vi "StepSysIDRealtime.vi"() -> ()   [LabVIEW 2011]
doc: "This VI was generated automatically using the FPGA Wizard. You can modify the VI normally."
uses:
  <vilib>/rvi/interface/nirviMethod/nirviMethod.xnode
  <vilib>/rvi/interface/nirviCloseFPGA/nirviCloseFPGA.xnode
  <vilib>/rvi/interface/nirviOpenFPGA/nirviOpenFPGA.xnode
  SysIDRealtime.lvlib
  <vilib>/rvi/interface/nirviReadWriteControl/nirviReadWriteControl.xnode
  <vilib>/rvi/errors/niLvFpgaAdjustHostInterfaceError.vi
  <vilib>/rvi/interface/Simulation/niFpgaSimulationCallBeginRW.vi
  NiFpgaLv.dll
  <vilib>/Utility/error.llb/Error Cluster From Error Code.vi
  <vilib>/Platform/TimedLoop/XDataNode/XDataNode.xnode
  <vilib>/Platform/TimedLoop/XDataNode/nitl_modes.ctl
  <vilib>/Platform/TimedLoop/XDataNode/XDNodeRunTimeDep.lvlib
  <vilib>/Platform/TimedLoop/XDataNode/wakeup.ctl
  <vilib>/Platform/TimedLoop/XDataNode/timing_clust.ctl
  <vilib>/Analysis/NI_AALBase.lvlib
  <vilib>/FPGAPlugInAG/Dynamic/niLvFpga_Reset_Dynamic.vi
  <vilib>/FPGAPlugInAG/Dynamic/niLvFpga_Run_Dynamic.vi
  <vilib>/FPGAPlugInAG/Dynamic/niLvFpga_Close_Dynamic.vi
  FPGA Bitfiles/PPDControlLab3_FPGATarget_SYSIDFPGA_8751AF80.lvbitx
  SYSID_FPGA.vi
  <vilib>/FPGAPlugInAG/sbRIO-9642/niLvFpga_Open_sbRIO-9642.vi
  <vilib>/rvi/interface/common/dynamic/niFpgaDynamicAddResources.vi
panel:
  out "Amp In":dbl[](graph)
  out "Amp Cpmmand":fxp<+/-,20,5>
  out "Iteration Duration":i64
  out "Position":i32[](graph)
  in  "Control Rate (ticks)":u32=800
  out "error":i32
  out "Waveform Graph":i32[](graph)
  in  "f2":dbl=0.5 format="%0.2f"
  in  "f1":dbl=1.0
  in  "amplitude":dbl=32767.0 format="%0.2f"
  in  "Period (us)":i64=400
  out "Finished Late? [i-1]":bool
  out "quad saved (Port0/DIO0,Port0/DIO1)":cluster{"Position":i32, "Index Count":u16}
  out "quad pos (Port0/DIO0,Port0/DIO1)":i32
  in  "AO (ModB/AO2)":fxp<+/-,20,5>
  in  "AO (ModB/AO1)":fxp<+/-,20,5>
  out "AI (ModA/AI0)":fxp<+/-,26,5> format="%.6g"
  out "Late? Latched":bool
  in  "Local Stop 0":bool
  in  "Start 0":bool
  in  "Loop Rate (Hz)":dbl=70000.0
  out "Calculated Rate (Hz)":dbl
  out "error out":errorcluster
  in  "Global Stop":bool
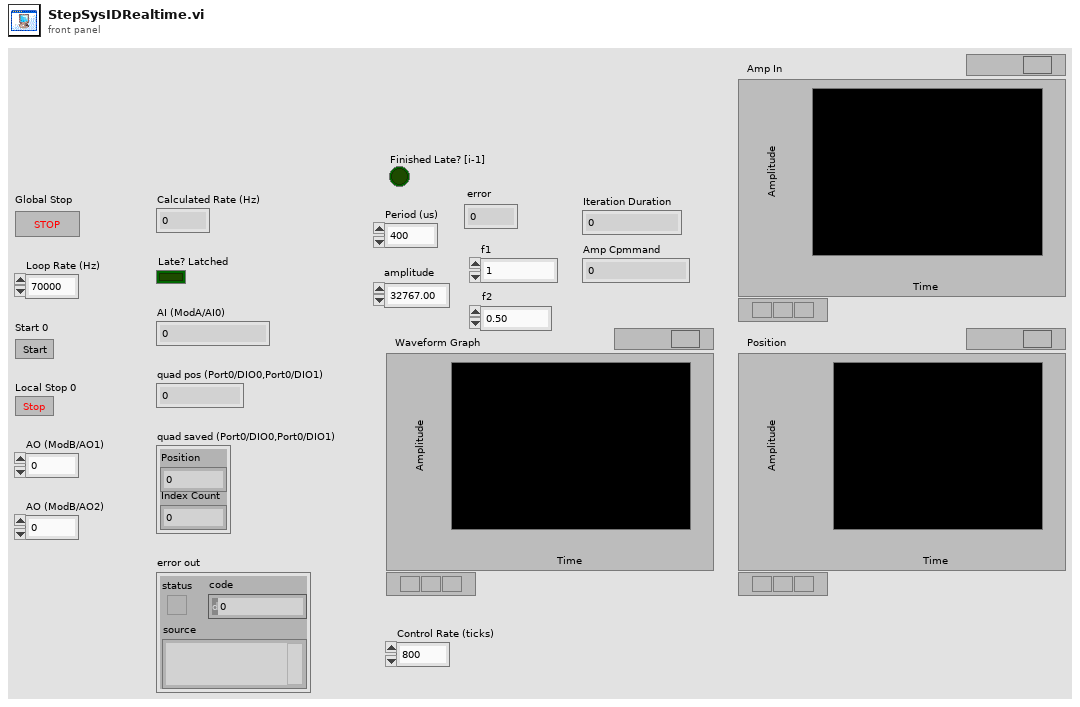
[diagram p1: front panel]
types:
  T1 = typedef "XDNodeRunTimeDep.lvlib/timing_clust.ctl" = cluster{"Expected End [f-1]":u64, "Actual End [f-1]":u64, "Finished Late? [f-1]":bool, "Expected End [i-1]":u64, "Actual End [i-1]":u64, "Finished Late? [i-1]":bool, "Expected Start [i]":u64, "Actual Start [i]":u64, "Expected Start [f]":u64, "Actual Start [f]":u64, "Source Name":string, "Structure Name":string, "Period":i64, "Deadline":i64, "Offset":i64, "Start":i64, "Priority":i32, "Timeout":i32, "Mode":T2, "Wakeup Reason":T3, "Error":errorcluster, "Source Type":string, "Secondary Source Type":string, "Global End Time":u64, "Global Start Time":u64, "Frame Duration":u64, "Iteration Duration":u64, "Assigned CPU":i32, "I/O Scan Engine Mode":u32}
  T2 = typedef "XDNodeRunTimeDep.lvlib/nitl_modes.ctl" = enum32{"No Change", "Process missed periods, maintain original phase", "Discard missed periods, maintain original phase", "Process missed periods, ignore original phase", "Discard missed periods, ignore original phase"}
  T3 = typedef "XDNodeRunTimeDep.lvlib/wakeup.ctl" = enum32{"Normal", "Aborted", "Asynchronous wakeup", "Timing source error", "Timed loop error", "Timeout"}
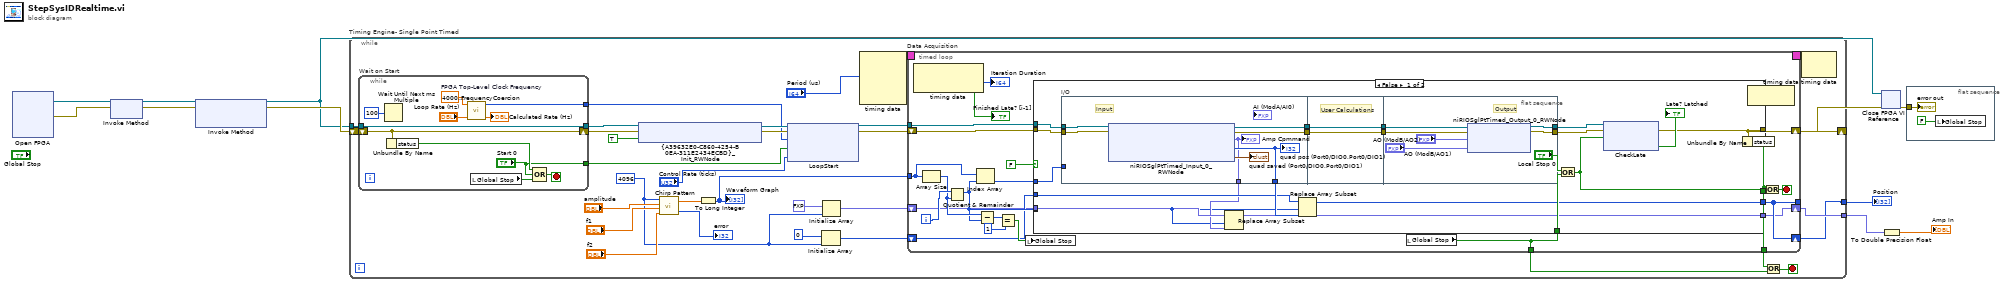
[diagram p0: block diagram]
diagram:
  n1 = xnode ("Open FPGA")() -> ("FPGA VI Reference Out"=w6:refnum<k20>, "error out"=w7:errorcluster)  [unwired: 2 in]
  n2 = xnode ("Invoke Method")("FPGA VI Reference In"=w6, "error in"=w7) -> ("FPGA VI Reference Out"=w10:refnum<k20>, "error out"=w11:errorcluster)
  n3 = xnode ("Invoke Method")("FPGA VI Reference In"=w10, "error in"=w11) -> ("FPGA VI Reference Out"=w8:refnum<k20>, "error out"=w9:errorcluster)  [unwired: 1 in]
  n4 = while "Timing Engine- Single Point Timed" {
    tunnel: w8 -> [w40]
    shift-right: [w39] -> w5
    shift-left: w9 -> [w43]
    tunnel: [w12] -> w3
    tunnel: [w13] -> w2
    stop <- w34 stop-if-true
    w15 = 4096 ("samples")
    n5 = while "Wait on Start" {
      tunnel: w40 -> [w121]
      tunnel: [w121] -> w38
      tunnel: [w113] -> w31
      tunnel: ["Start 0"] -> w30
      shift-right: [w115] -> w37
      shift-left: w43 -> [w115]
      stop <- w122 stop-if-true
      w116 = 40000000.0  # FPGA Top-Level Clock Frequency
      n6 = Wait Until Next ms Multiple(millisecond multiple=u32 100) -> ()  [unwired: 1 out]
      n7 = Unbundle By Name(w115) -> ("status"=w114:bool)
      n8 = call "FrequencyCoercion.vi"("Loop Rate (Hz)"="Loop Rate (Hz)", "FPGA Top-Level Clock Frequency"=w116) -> ("Actual Rate (Hz)"=→"Calculated Rate (Hz)":dbl, "FPGA Ticks"=w113:u32)  [unwired: 2 in]
      n9 = local read "Global Stop"() -> (w119:bool)
      n10 = Compound Arithmetic op=OR(w114, "Start 0", w119) -> (w122:bool)
    }
    n11 = xnode ("{A39632E0-C860-4254-B0EA-311E2434ECBD}_Init_RWNode")("FPGA VI Reference In"=w38, "error in"=w37, "quad reset (Port0/DIO0,Port0/DIO1)"=TRUE ("const")) -> ("FPGA VI Reference Out"=w32:refnum<k20>, "error out"=w36:errorcluster)
    n12 = call <vilib>:"Chirp Pattern.vi"("f2"="f2", "f1"="f1", "amplitude"="amplitude", "samples"=w15) -> ("error"=→"error":i32, "Chirp Pattern"=w21:dbl[])
    n13 = To Long Integer(number=w21) -> (32bit integer=w20:i32[])
    "Waveform Graph" <- w20
    n14 = xnode ("LoopStart")("FPGA VI Reference In"=w32, "error in"=w36, "Loop Rate (Ticks)"=w31, "Start 0"=w30, "Control Rate (ticks)"="Control Rate (ticks)") -> ("FPGA VI Reference Out"=w42:refnum<k20>, "error out"=w41:errorcluster)
    n15 = Initialize Array(0 ("quad pos (Port0/DIO0,Port0/DIO1)"), w15) -> (w17:i32[])
    n16 = Initialize Array(fxp<+/-,20,5> 0.0 ("Amp Cpmmand"), w15) -> (w14:fxp<+/-,20,5>[])
    n17 = node-c288("Period (us)") -> (w28:T1)  [unwired: 3 in]
    n18 = timed-loop "Data Acquisition" {
      tunnel: w42 -> [w60]
      tunnel: [w62] -> w35
      tunnel: [w61] -> w33
      shift-right: [w65] -> w39
      shift-left: w41 -> [w59]
      timing: w28 -> [_]
      timing-out: [_] -> w27
      tunnel: w20 -> [w55]
      tunnel: [w45] -> _
      shift-right: [w44] -> w13
      shift-left: w14 -> [w46]
      shift-right: [w45] -> w12
      shift-left: w17 -> [w48]
      i -> [w56]
      stop <- w63 stop-if-true
      n19 = node-c288() -> (→"Finished Late? [i-1]":bool, →"Iteration Duration":i64)  [unwired: 1 in]
      n20 = Array Size(array=w55) -> (size(s)=w53:i32)
      n21 = Quotient & Remainder(x=w56, y=w53) -> (x-y*floor(x/y)=w49:i32)  [unwired: 1 out]
      n22 = Index Array(array=w55, index=w49) -> (element=w54:i32)
      n23 = Subtract(x=w53, y=w49) -> (x-y=w52:i32)
      n24 = Equal?(x=w52, y=1) -> (x = y?=w50:bool)
      n25 = local write "Global Stop"(w50) -> ()
      n26 = local read "Global Stop"() -> (w62:bool)
      n27 = case "Timeout" shown="False" FALSE {
        tunnel: w60 -> [w85 _]
        tunnel: w59 -> [w84 w107]
        tunnel: [w78 w107] -> w65
        tunnel: [w80 w106] -> w64
        tunnel: w62 -> [w81 w106]
        tunnel: w54 -> [w77 _]
        tunnel: w49 -> [w71 _]
        tunnel: w48 -> [w75 _]
        tunnel: [w74 _] -> w45
        tunnel: w46 -> [w73 _]
        tunnel: [w70 _] -> w44
        frame False {
          n28 = flat-sequence "I/O" {
            tunnel: w85 -> [w95]
            tunnel: w84 -> [w97]
            tunnel: [w96] -> w90
            tunnel: [w94] -> w87
            tunnel: w77 -> [_]
            tunnel: [w92] -> w76
            tunnel: [w91] -> w72
            tunnel: [w99] -> w89
            tunnel: w90 -> [w98]
            tunnel: w87 -> [w99]
            tunnel: [w98] -> w88
            tunnel: [w104] -> w83
            tunnel: [w102] -> w86
            tunnel: w89 -> [w103]
            tunnel: w88 -> [w105]
            frame #0 {
              # "Input"
              n29 = xnode ("niRIOSglPtTimed_Input_0_RWNode")("FPGA VI Reference In"=w95, "error in"=w97) -> ("FPGA VI Reference Out"=w94:refnum<k20>, "error out"=w96:errorcluster, "Amp Cpmmand"=w91:fxp<+/-,20,5>, "quad pos (Port0/DIO0,Port0/DIO1)"=w92:i32, "quad saved (Port0/DIO0,Port0/DIO1)"=→"quad saved (Port0/DIO0,Port0/DIO1)":cluster{"Position":i32, "Index Count":u16})
              "quad pos (Port0/DIO0,Port0/DIO1)" <- w92
              "Amp Cpmmand" <- w91
            }
            frame #1 {
              # "User Calculations"
            }
            frame #2 {
              # "Output"
              n30 = xnode ("niRIOSglPtTimed_Output_0_RWNode")("FPGA VI Reference In"=w103, "error in"=w105, "AO (ModB/AO1)"="AO (ModB/AO1)", "AO (ModB/AO2)"="AO (ModB/AO2)") -> ("FPGA VI Reference Out"=w102:refnum<k20>, "error out"=w104:errorcluster)
            }
          }
          n31 = Replace Array Subset(array=w73, new element=w72, index=w71) -> (w70:fxp<+/-,20,5>[])
          n32 = Replace Array Subset(array=w75, new element=w76, index=w71) -> (w74:i32[])
          n33 = Or(x="Local Stop 0", y=w81) -> (x .or. y?=w80:bool)
          n34 = xnode ("CheckLate")("FPGA VI Reference In"=w86, "error in"=w83, "Local Stop 0"=w80) -> ("error out"=w78:errorcluster, "Late? Latched"=→"Late? Latched":bool)  [unwired: 1 out]
        }
        frame True {
          # "Timeout waiting for an interrupt. This case checks the state of the global stop.\nIf global stop is not set, then loop around to wait for an interrupt again."
        }
      }
      n35 = Unbundle By Name(w65) -> ("status"=w61:bool)
      n36 = node-c288() -> ()  [unwired: 1 in, 1 out]
      n37 = Or(x=w61, y=w64) -> (x .or. y?=w63:bool)
    }
    n38 = Or(x=w33, y=w35) -> (x .or. y?=w34:bool)
    n39 = node-c288(w27) -> ()  [unwired: 1 out]
  }
  "Position" <- w3
  n40 = xnode ("Close FPGA VI Reference")("FPGA VI Reference In"=w8, "error in"=w5) -> ("error out"=w4:errorcluster)
  n41 = To Double Precision Float(number=w2) -> (double precision float=→"Amp In":dbl[])
  n42 = flat-sequence {
    tunnel: w4 -> [w124]
    frame #0 {
      n43 = local write "Global Stop"(FALSE ("Global Stop")) -> ()
      "error out" <- w124
    }
  }
